vi "Entradas.vi"(11 "Class 2.lvclass":refnum<class "Class 2.lvclass">) -> (3 "Class 2.lvclass 2":refnum<class "Class 2.lvclass">)   [LabVIEW 2019, in "Class 2.lvclass"]
uses:
  Class 2.lvclass
  Class 2.lvclass/Class 2.ctl
  Datos Out.vi
  Datos In.vi
panel:
  out "current time":u32
  out "current time 2":u32
  in  "PRUEBA DE CONTACTOS":string(combo)
  in  "PRUEBA DE DISTANCIA":string(combo)
  in  "PRUEBA DE TENSION":string(combo)
  in  "ENTRADAS.HOME C2":bool
  in  "ENTRADAS.PIEZA EN EL NIDO":bool
  in  "ENTRADAS.SMAC TOMA DE MUESTRA":bool
  in  "ENTRADAS.SMAC APROXIMACION":bool
  in  "ENTRADAS.SMAC AVANCE SEGURO":bool
  in  "ENTRADAS.SMAC HOME":bool
  in  "ENTRADAS.AVANCE C2":bool
  in  "ENTRADAS.AVANCE C1":bool
  in  "ENTRADAS.HOME C1":bool
  in  "ENTRADAS.BIMANUAL 2":bool
  in  "ENTRADAS.BIMANUAL 1":bool
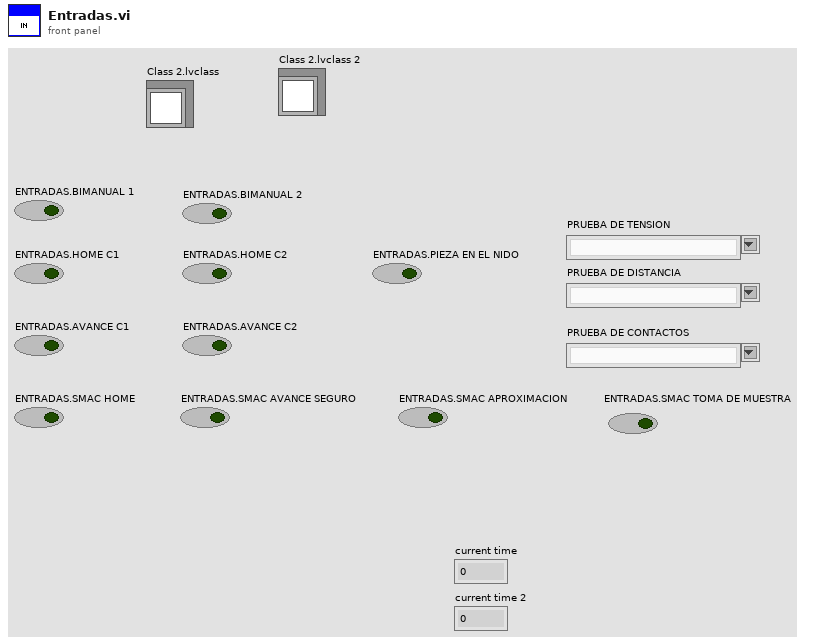
[diagram p1: front panel]
types:
  T1 = cluster{"Test":bool, "CILINDRO _1":bool, "CILINDRO _2":bool, "SMAC_RETORNANDO":bool, "SMAC_AVANZANDO":bool, "MANUAL":bool, "EST_1":bool, "EST_2":bool, "EST_3":bool, "MOVER A ORIGEN":bool, "RESET":bool, "PARO":bool, "INICIO":bool, "DATA_CONTROL":cluster{"ESTACION_1":cluster{"ACEPTADA":bool, "MAXIMO":dbl, "MINIMO":dbl, "LECTURA":dbl}, "ESTACION_2":cluster{"ACEPTADA":bool, "MAXIMO":dbl, "MINIMO":dbl, "LECTURA":dbl}, "ESTACION_3":cluster{"ACEPTADA":bool, "MAXIMO":dbl, "MINIMO":dbl, "LECTURA":dbl}}}
  T2 = cluster{"Numeric":dbl, "VALOR DE DISTANCIA":dbl, "VALOR DE TENSION":dbl}
  T3 = cluster{"DATO GAP":string, "DATO TENSION":string, "mensajes usuario":string}
  T4 = cluster{"SALIDAS.CILINDRO 1":bool, "SALIDAS.CILINDRO 2":bool, "SALIDAS.SEMAC RETORNANDO":bool, "SALIDAS.SAMAC AVANZANDO":bool, "Auto(off)/Manual(on)":bool, "HOME_CILINDRO_1":bool, "HOME_CILINDRO_2":bool, "AVANCE_CILINDRO_1":bool, "AVANCE_CILINDRO_2":bool, "PIEZA_EN_NIDO":bool, "BIMANUAL 2":bool, "BIMANUAL1":bool, "SIN CAMBIOS":bool, "CON  CAMBIOS":bool, "TESTER":bool, "MAQUINA EN ORIGEN":bool, "FALLA PRESENTE":bool}
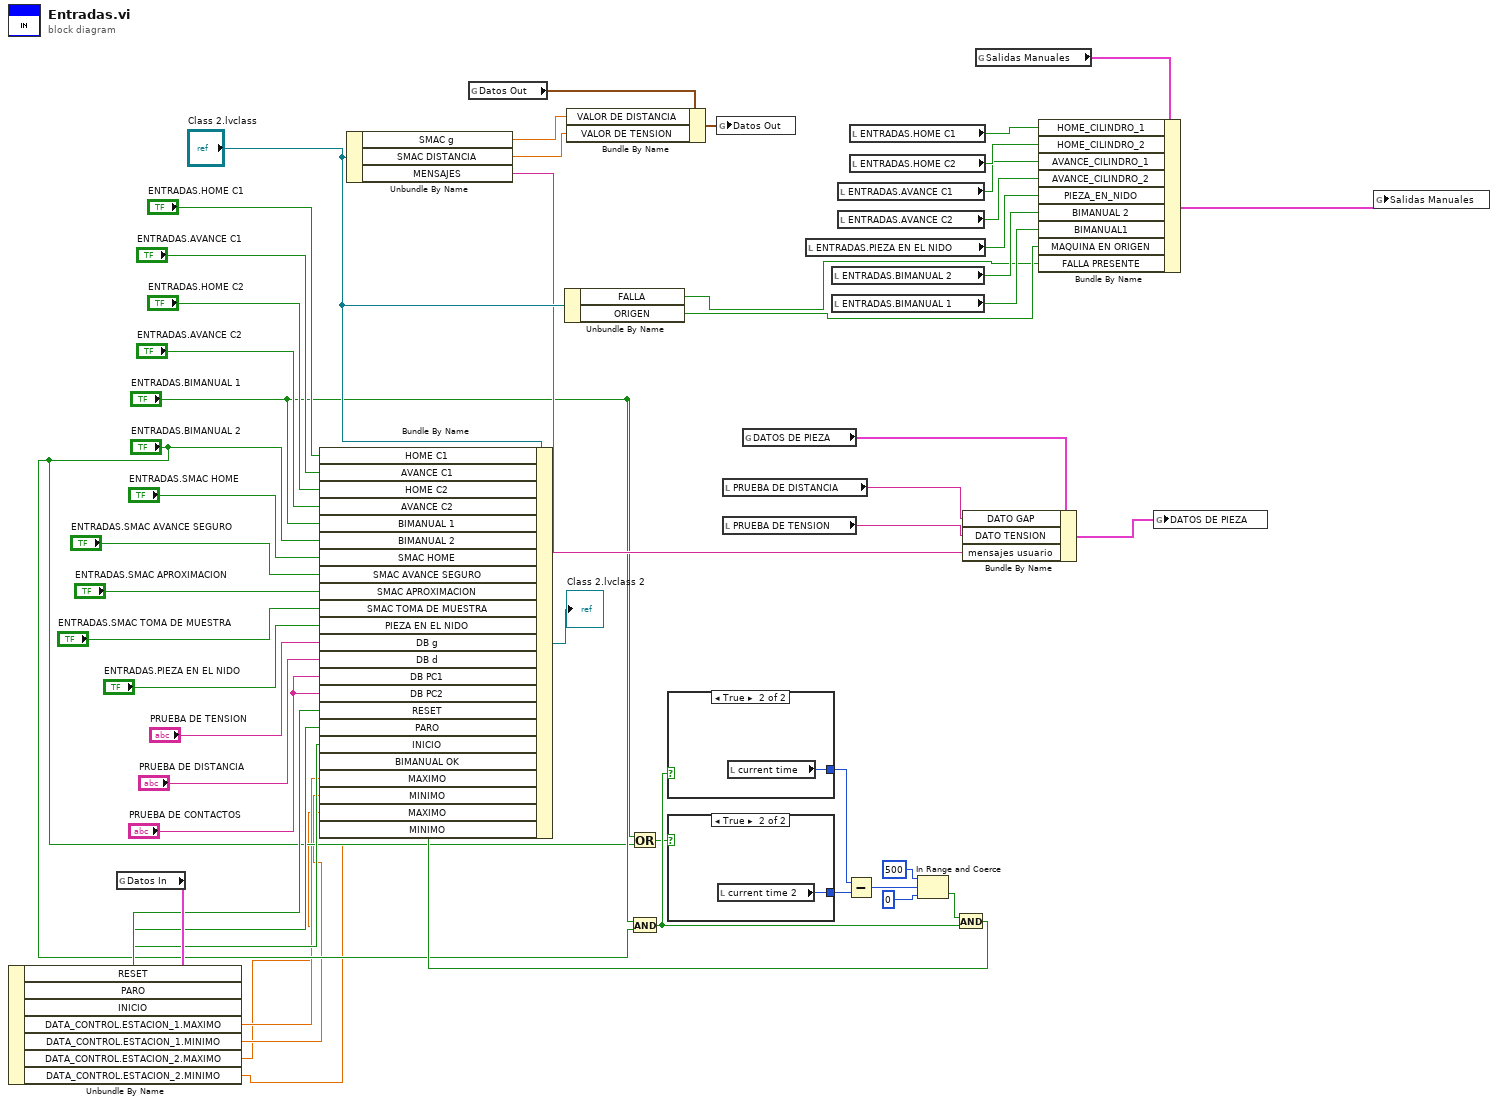
[diagram p0: block diagram]
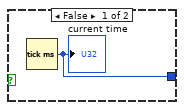
[diagram p2: hidden frame]
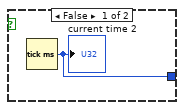
[diagram p3: hidden frame]
diagram:
  n1 = global read "Datos In.vi" "Datos In"() -> (w28:T1)
  n2 = Unbundle By Name(w28) -> ("RESET"=w27:bool, "PARO"=w26:bool, "INICIO"=w16:bool, "DATA_CONTROL.ESTACION_1.MAXIMO"=w4:dbl, "DATA_CONTROL.ESTACION_1.MINIMO"=w3:dbl, "DATA_CONTROL.ESTACION_2.MAXIMO"=w2:dbl, "DATA_CONTROL.ESTACION_2.MINIMO"=w1:dbl)
  n3 = Unbundle By Name("Class 2.lvclass") -> ("SMAC g"=w30:dbl, "SMAC DISTANCIA"=w29:dbl, "MENSAJES"=w17:string)
  n4 = global read "Datos Out.vi" "Datos Out"() -> (w32:T2)
  n5 = Unbundle By Name("Class 2.lvclass") -> ("FALLA"=w22:bool, "ORIGEN"=w23:bool)
  n6 = Bundle By Name(cluster=w32, "VALOR DE DISTANCIA"=w30, "VALOR DE TENSION"=w29) -> (w31:T2)
  n7 = Or(x="ENTRADAS.BIMANUAL 1", y="ENTRADAS.BIMANUAL 2") -> (x .or. y?=w11:bool)
  n8 = And(x="ENTRADAS.BIMANUAL 1", y="ENTRADAS.BIMANUAL 2") -> (x .and. y?=w15:bool)
  n9 = case shown="True" w15 {
    tunnel: [w54 w55] -> w10
    frame False {
      n10 = Tick Count (ms)() -> (millisecond timer value=w54:u32)
      "current time" <- w54
    }
    frame True {
      n11 = local read "current time"() -> (w55:u32)
    }
  }
  n12 = case shown="True" w11 {
    tunnel: [w56 w57] -> w9
    frame False {
      n13 = Tick Count (ms)() -> (millisecond timer value=w56:u32)
      "current time 2" <- w56
    }
    frame True {
      n14 = local read "current time 2"() -> (w57:u32)
    }
  }
  n15 = global write "Datos Out.vi" "Datos Out"(w31) -> ()
  n16 = local read "PRUEBA DE DISTANCIA"() -> (w19:string)
  n17 = local read "PRUEBA DE TENSION"() -> (w18:string)
  n18 = global read "Datos Out.vi" "DATOS DE PIEZA"() -> (w21:T3)
  n19 = local read "ENTRADAS.PIEZA EN EL NIDO"() -> (w34:bool)
  n20 = local read "ENTRADAS.BIMANUAL 2"() -> (w33:bool)
  n21 = local read "ENTRADAS.BIMANUAL 1"() -> (w25:bool)
  n22 = local read "ENTRADAS.AVANCE C1"() -> (w36:bool)
  n23 = local read "ENTRADAS.AVANCE C2"() -> (w35:bool)
  n24 = Subtract(x=w10, y=w9) -> (x-y=w12:u32)
  n25 = local read "ENTRADAS.HOME C1"() -> (w38:bool)
  n26 = local read "ENTRADAS.HOME C2"() -> (w37:bool)
  n27 = In Range and Coerce(upper limit=u32 500, x=w12, lower limit=u32 0) -> (In Range?=w14:bool)  [unwired: 1 out]
  n28 = And(x=w14, y=w15) -> (x .and. y?=w7:bool)
  n29 = Bundle By Name(cluster="Class 2.lvclass", "HOME C1"="ENTRADAS.HOME C1", "AVANCE C1"="ENTRADAS.AVANCE C1", "HOME C2"="ENTRADAS.HOME C2", "AVANCE C2"="ENTRADAS.AVANCE C2", "BIMANUAL 1"="ENTRADAS.BIMANUAL 1", "BIMANUAL 2"="ENTRADAS.BIMANUAL 2", "SMAC HOME"="ENTRADAS.SMAC HOME", "SMAC AVANCE SEGURO"="ENTRADAS.SMAC AVANCE SEGURO", "SMAC APROXIMACION"="ENTRADAS.SMAC APROXIMACION", "SMAC TOMA DE MUESTRA"="ENTRADAS.SMAC TOMA DE MUESTRA", "PIEZA EN EL NIDO"="ENTRADAS.PIEZA EN EL NIDO", "DB g"="PRUEBA DE TENSION", "DB d"="PRUEBA DE DISTANCIA", "DB PC1"="PRUEBA DE CONTACTOS", "DB PC2"="PRUEBA DE CONTACTOS", "RESET"=w27, "PARO"=w26, "INICIO"=w16, "BIMANUAL OK"=w7, "MAXIMO"=w4, "MINIMO"=w3, "MAXIMO"=w2, "MINIMO"=w1) -> (→"Class 2.lvclass 2":refnum<class "Class 2.lvclass">)
  n30 = Bundle By Name(cluster=w21, "DATO GAP"=w19, "DATO TENSION"=w18, "mensajes usuario"=w17) -> (w20:T3)
  n31 = global read "Datos Out.vi" "Salidas Manuales"() -> (w40:T4)
  n32 = Bundle By Name(cluster=w40, "HOME_CILINDRO_1"=w38, "HOME_CILINDRO_2"=w37, "AVANCE_CILINDRO_1"=w36, "AVANCE_CILINDRO_2"=w35, "PIEZA_EN_NIDO"=w34, "BIMANUAL 2"=w33, "BIMANUAL1"=w25, "MAQUINA EN ORIGEN"=w23, "FALLA PRESENTE"=w22) -> (w39:T4)
  n33 = global write "Datos Out.vi" "DATOS DE PIEZA"(w20) -> ()
  n34 = global write "Datos Out.vi" "Salidas Manuales"(w39) -> ()
